vi "write TBM configuration.vi"(8 "error in":errorcluster, 10 "configuration":refnum<class "TBM configuration.lvclass">, 11 "Getting Started IO editor node in":refnum<class "UI Reference editor node.lvclass">) -> (0 "error out":errorcluster, 3 "Getting Started IO editor node out":refnum<class "UI Reference editor node.lvclass">)   [LabVIEW 2013, in "UI Reference editor node.lvclass"]
uses:
  UI Reference editor node.lvclass
  <vilib>/NI/Tag Bus Module Framework/root configuration/TBM configuration.lvclass
  module/configuration/UI Reference configuration.lvclass
  UI Reference editor node.lvclass/UI Reference editor node.ctl
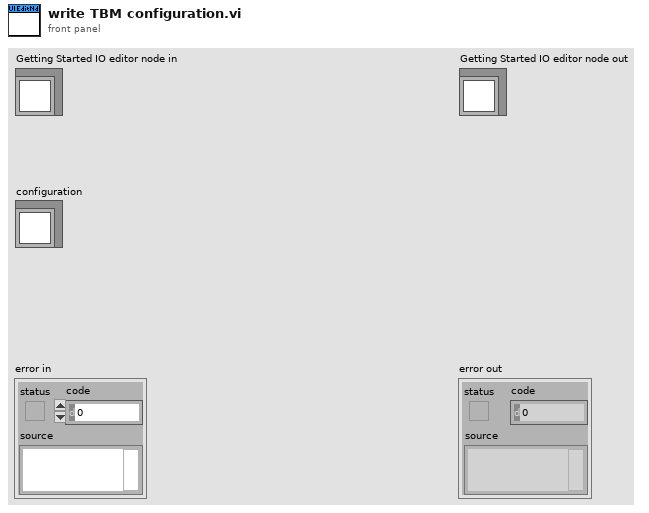
[diagram p1: front panel]
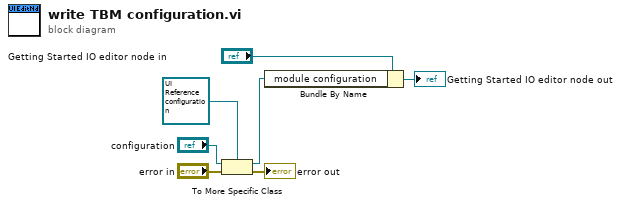
[diagram p0: block diagram]
diagram:
  n1 = To More Specific Class(target class=refnum<class "UI Reference configuration.lvclass"> refnum ("module configuration"), reference="configuration", error in="error in") -> (specific class reference=w1:refnum<class "UI Reference configuration.lvclass">, error out=→"error out":errorcluster)
  n2 = Bundle By Name(cluster="Getting Started IO editor node in", "module configuration"=w1) -> (→"Getting Started IO editor node out":refnum<class "UI Reference editor node.lvclass">)
